vi "type_01_int8_one_segment.vi"() -> ()   [LabVIEW 2010]
panel:
  out "error out":errorcluster
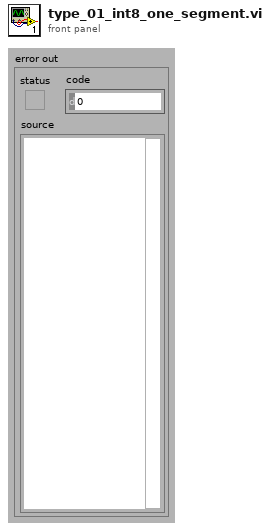
[diagram p1: front panel]
types:
  T1 = enum16{"open", "open or create", "create or replace", "create", "open (read-only)"}
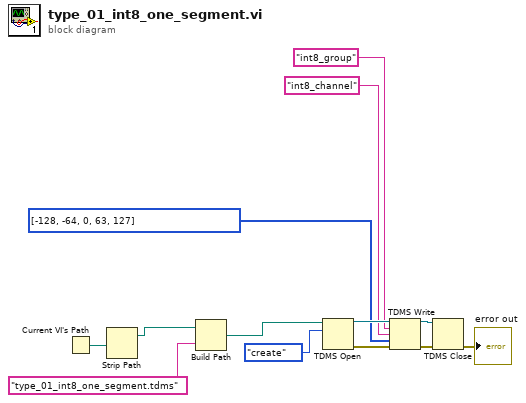
[diagram p0: block diagram]
diagram:
  n1 = Current VI's Path() -> (path=w5:path)
  n2 = Strip Path(path=w5) -> (stripped path=w4:path)  [unwired: 1 out]
  n3 = Build Path(base path=w4, name or relative path="type_01_int8_one_segment.tdms") -> (appended path=w2:path)
  n4 = TDMS Open(10:T1."create" ("operation (0:open)"), 11:w2) -> (0:w13:errorcluster, 3:w12:refnum<k34>)  [unwired: 4 in]
  n5 = TDMS Write(0:w12, 5:"int8_group" ("group name in (Untitled)"), 7:"int8_channel" ("channel name(s) in (Untitled)"), 9:i8[] [-128, -64, 0, 63, 127], 11:w13) -> (4:w8:refnum<k34>, 15:w7:errorcluster)  [unwired: 1 in, 2 out]
  n6 = TDMS Close(8:w7, 11:w8) -> (0:→"error out":errorcluster)  [unwired: 1 out]
